vi "MuC_Sample_Rate.vi"(1 "N smpls":i32, 2 "Frequency / Hz":dbl) -> (0 "Sample Period / us":i32)   [LabVIEW 2019]
doc: "Compute value of sample rate based on known operating frequency and desired number of samples per\nperiod. \n\nSample Rate must be higher than frequency of signal being sampled. \n\nR. Sheehan 8 - 11 - 2018\n\nOriginally written for Tektronix High-speed scope, updated for use with Arduino Micro\n\nR. Sheehan 27 - 1 - 2021"
panel:
  out "Sample Period / ms":dbl
  out "Sample Rate / Hz":dbl
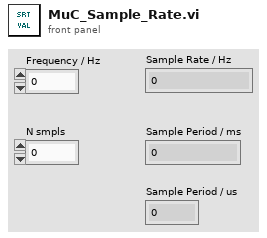
[diagram p1: front panel]
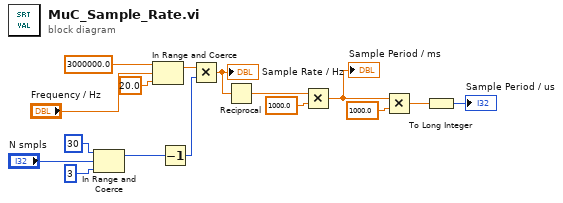
[diagram p0: block diagram]
diagram:
  n1 = In Range and Coerce(upper limit=30, x="N smpls", lower limit=3) -> (coerced(x)=w8:i32)  [unwired: 1 out]
  n2 = In Range and Coerce(upper limit=3000000.0, x="Frequency / Hz", lower limit=20.0) -> (coerced(x)=w9:dbl)  [unwired: 1 out]
  n3 = Decrement(x=w8) -> (x-1=w6:i32)
  n4 = Multiply(x=w9, y=w6) -> (x*y=w16:dbl)
  "Sample Rate / Hz" <- w16
  n5 = Reciprocal(x=w16) -> (1/x=w15:dbl)
  n6 = Multiply(x=w15, y=1000.0) -> (x*y=w12:dbl)
  "Sample Period / ms" <- w12
  n7 = Multiply(x=w12, y=1000.0) -> (x*y=w11:dbl)
  n8 = To Long Integer(number=w11) -> (32bit integer=→"Sample Period / us":i32)
